vi "Read Required Keys - Type.vi"() -> (2 "Required Keys":string[](array[string]))   [LabVIEW 2019, in "Configuration.lvlib" / "Configuration.lvclass"]
uses:
  Configuration.lvclass
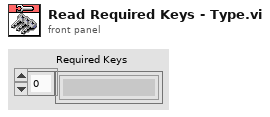
[diagram p1: front panel]
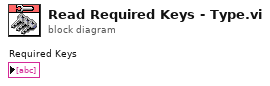
[diagram p0: block diagram]
diagram:
